vi "SeCrTS-DD Queue Data log module.vi"(8 "error in":errorcluster) -> (0 "error out":errorcluster)   [LabVIEW 2022 SP3]
uses:
  Control/SeCrTS-Datalog enumDD.ctl
  Globals/SeCrTS-DD globals.vi
panel:
  out "x":u32
  out "x-y":dbl
  out "Restart":bool
  out "Log health":bool
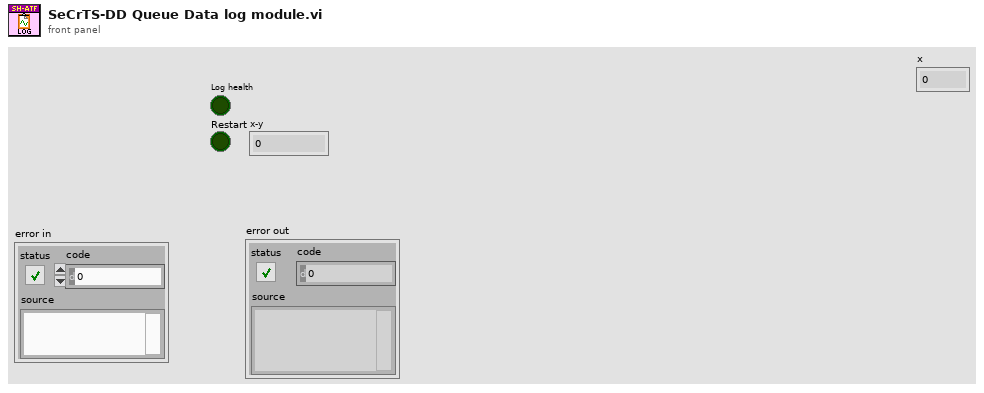
[diagram p1: front panel]
types:
  T1 = cluster{"Log In Progress?":bool, "Log Start Time":timestamp, "Analog Queues":refnum<queue>[], "Digital Queues":refnum<queue>[], "tdms file ref":refnum<k34>}
  T2 = typedef "SeCrTS-Datalog enumDD.ctl" = enum16{"Initialize", "Poll", "Create file", "log Analog", "log Digital", "Flush Queues", "Close file", "Error", "Exit"}
  T3 = enum16{"open", "open or create", "create or replace", "create", "open (read-only)"}
  T4 = cluster{"Datalog path":path, "Configuration path":path, "Signal list path":path, "Sub vi's":path, "Authentication":path}
  T5 = cluster{"Channel names":cluster{"AI_C_Data P":string[], "AI_V_Data P":string[], "AO_Data P":string[], "DO_Data P":string[], "ACC_Data P":string[], "TC Data P":string[], "Drive_A_C":string[], "Drive_A_D":string[], "AI_C_Data S":string[], "DO_Data S":string[]}, "DI Names":cluster{"Di P":string[], "Di S":string[]}}
  T6 = cluster{"AI_C_Data P":string[], "AI_V_Data P":string[], "AO_Data P":string[], "DO_Data P":string[], "ACC_Data P":string[], "TC Data P":string[], "Drive_A_C":string[], "Drive_A_D":string[], "AI_C_Data S":string[], "DO_Data S":string[]}
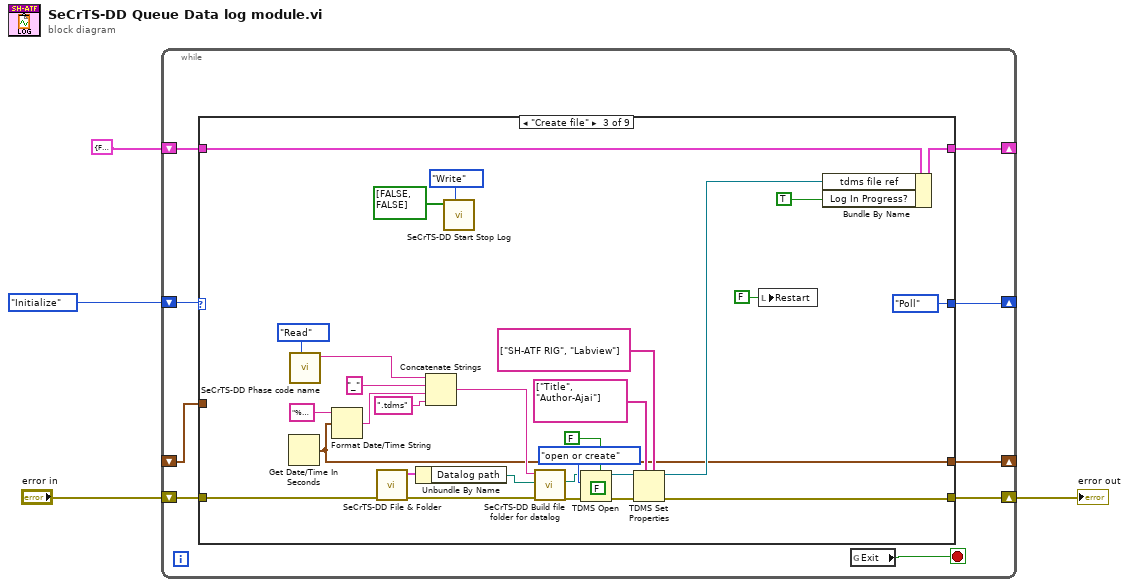
[diagram p0: block diagram]
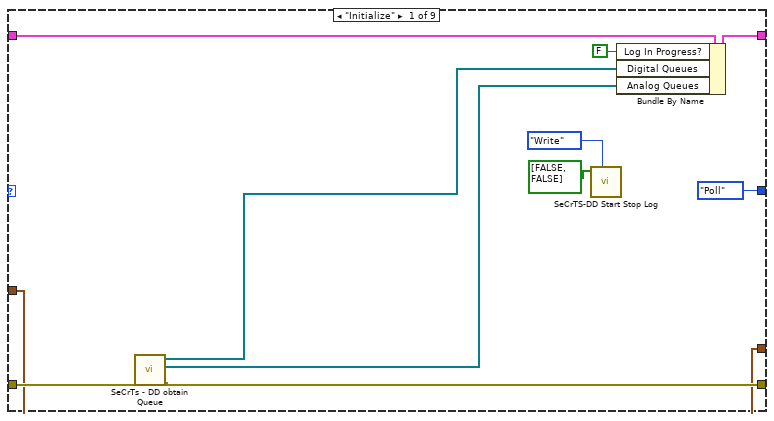
[diagram p2: hidden frame]
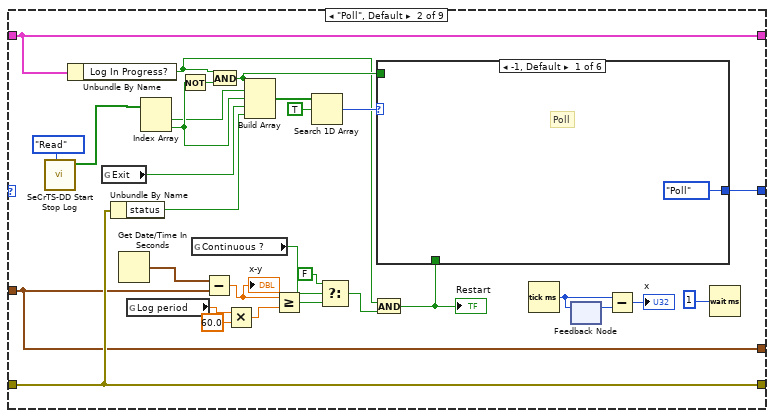
[diagram p3: hidden frame]
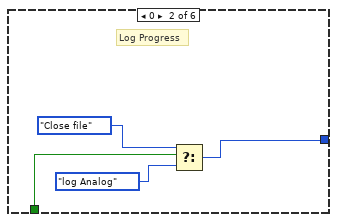
[diagram p4: hidden frame]
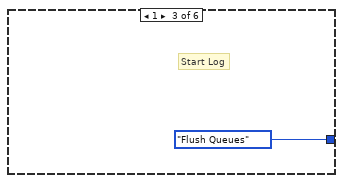
[diagram p5: hidden frame]
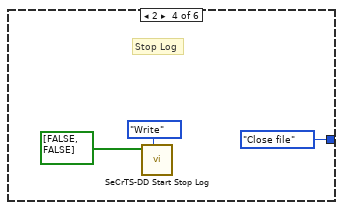
[diagram p6: hidden frame]
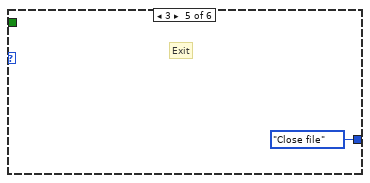
[diagram p7: hidden frame]
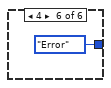
[diagram p8: hidden frame]
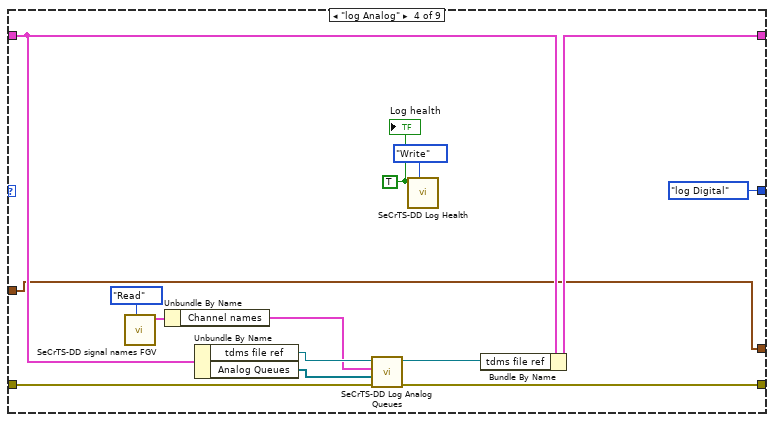
[diagram p9: hidden frame]
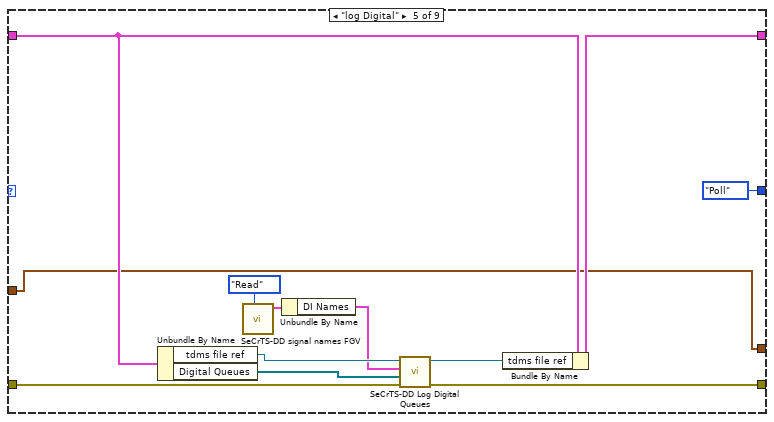
[diagram p10: hidden frame]
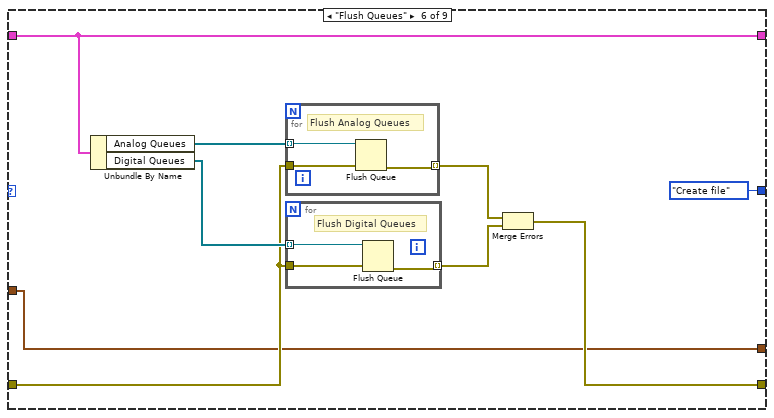
[diagram p11: hidden frame]
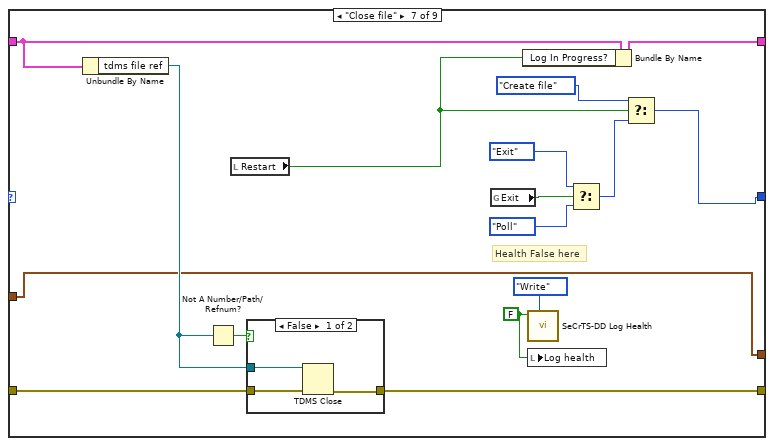
[diagram p12: hidden frame]
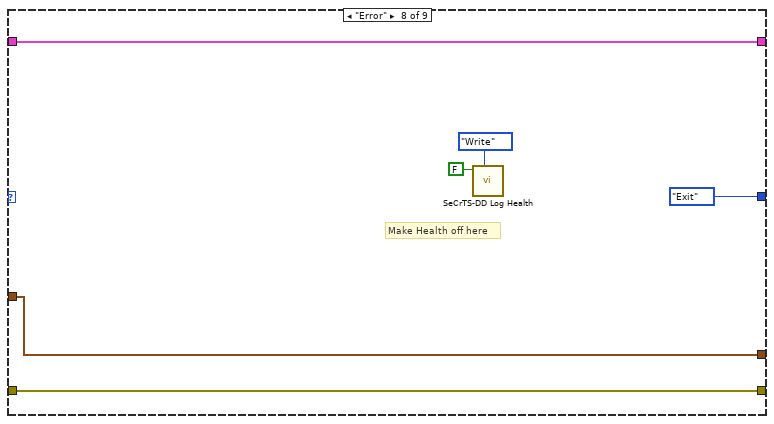
[diagram p14: hidden frame]
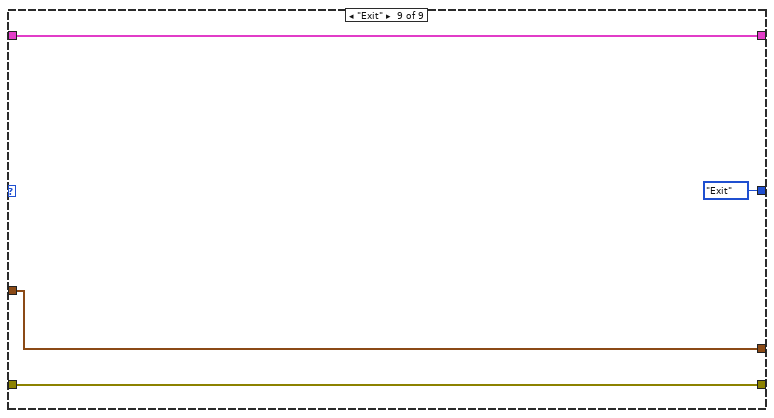
[diagram p15: hidden frame]
diagram:
  n1 = while {
    shift-right: [w8] -> _
    shift-left: SeCrTS-Datalog_enumDD."Initialize" -> [w13]
    shift-right: [w10] -> _
    shift-left: T1 {"Log In Progress?"=FALSE, "Log Start Time"=timestamp(0 s since 1904-01-01), "Analog Queues"=[], "Digital Queues"=[], "tdms file ref"=refnum} -> [w11]
    shift-right: [w9] -> w1
    shift-left: "error in" -> [w12]
    shift-right: [w5] -> _
    shift-left: _ -> [w6]
    stop <- w7 stop-if-true
    n2 = case shown="\"Create file\"" w13 {
      tunnel: w12 -> [w23 w48 w89 w105 w119 w125 w147 w159 w164]
      tunnel: w11 -> [w24 w54 w78 w107 w117 w128 w148 w161 w165]
      tunnel: [w22 w54 w77 w102 w114 w128 w149 w161 w165] -> w10
      tunnel: [w18 w48 w74 w104 w118 w122 w146 w159 w164] -> w9
      tunnel: [SeCrTS-Datalog_enumDD."Poll" w49 SeCrTS-Datalog_enumDD."Poll" SeCrTS-Datalog_enumDD."log Digital" SeCrTS-Datalog_enumDD."Poll" SeCrTS-Datalog_enumDD."Create file" w136 SeCrTS-Datalog_enumDD."Exit" SeCrTS-Datalog_enumDD."Exit"] -> w8
      tunnel: w6 -> [w16 w38 _ w95 w109 w121 w140 w156 w162]
      tunnel: [w16 w38 w68 w95 w109 w121 w140 w156 w162] -> w5
      frame "Initialize" {
        n3 = call "SeCrTs - DD obtain Queue.vi"("error in"=w23) -> ("error out"=w18:errorcluster, "AI_V_Data P\nAI_C_Data P\nAO_Data P\nDO_Data P\nACC_Data P\nTC Data P\nDrive_A_C \nDrive_A_D\nAI_C_Data S\nDO_Data S\nAI_V_Rms_P"=w19:refnum<queue>[], "DI P\nDI S"=w20:refnum<queue>[])  [unwired: 8 in]
        n4 = call "SeCrTS-DD Start Stop Log.vi"("Enum"=enum16{"Read", "Write"}."Write", "Start Stop log"=bool[] [FALSE, FALSE]) -> ()  [unwired: 8 in, 2 out]
        n5 = Bundle By Name(cluster=w24, "Log In Progress?"=FALSE, "Digital Queues"=w20, "Analog Queues"=w19) -> (w22:T1)
      }
      frame "Poll", Default {
        n6 = call "SeCrTS-DD Start Stop Log.vi"("Enum"=enum16{"Read", "Write"}."Read") -> ("Start Stop log R"=w34:bool[])  [unwired: 9 in, 1 out]
        n7 = Unbundle By Name(w54) -> ("Log In Progress?"=w28:bool)
        n8 = global read "SeCrTS-DD globals.vi" "Exit"() -> (w44:bool)
        n9 = Unbundle By Name(w48) -> ("status"=w53:bool)
        n10 = Get Date/Time In Seconds() -> (seconds since 1Jan1904=w40:timestamp)
        n11 = global read "SeCrTS-DD globals.vi" "Log period"() -> (w27:dbl)
        n12 = Index Array(array=w34) -> (element #1=w45:bool, element #2=w46:bool)  [unwired: 2 in]
        n13 = Not(x=w46) -> (.not. x?=w47:bool)
        n14 = global read "SeCrTS-DD globals.vi" "Continuous ?"() -> (w32:bool)
        n15 = Subtract(x=w40, y=w38) -> (x-y=w41:dbl)
        "x-y" <- w41
        n16 = And(x=w28, y=w47) -> (x .and. y?=w42:bool)
        n17 = Multiply(x=w27, y=60.0) -> (x*y=w25:dbl)
        n18 = Build Array(w42, w45, w46, w44, w53) -> (w52:bool[])
        n19 = Greater Or Equal?(x=w41, y=w25) -> (x >= y?=w31:bool)
        n20 = Search 1D Array(1D array=w52, element=TRUE) -> (index of element=w50:i32)  [unwired: 1 in]
        n21 = Select(t=FALSE, s=w32, f=w31) -> (s? t:f=w29:bool)
        n22 = And(x=w28, y=w29) -> (x .and. y?=w39:bool)
        "Restart" <- w39
        n23 = case shown="-1, Default" w50 {
          tunnel: [SeCrTS-Datalog_enumDD."Poll" w56 SeCrTS-Datalog_enumDD."Flush Queues" SeCrTS-Datalog_enumDD."Close file" SeCrTS-Datalog_enumDD."Close file" SeCrTS-Datalog_enumDD."Error"] -> w49
          tunnel: w42 -> [_ _ _ _ _ _]
          tunnel: w39 -> [_ w59 _ _ _ _]
          frame -1, Default {
            # "Poll"
          }
          frame 0 {
            # "Log Progress"
            n24 = Select(t=SeCrTS-Datalog_enumDD."Close file", s=w59, f=SeCrTS-Datalog_enumDD."log Analog") -> (s? t:f=w56:T2)
          }
          frame 1 {
            # "Start Log"
          }
          frame 2 {
            # "Stop Log"
            n25 = call "SeCrTS-DD Start Stop Log.vi"("Enum"=enum16{"Read", "Write"}."Write", "Start Stop log"=bool[] [FALSE, FALSE]) -> ()  [unwired: 8 in, 2 out]
          }
          frame 3 {
            # "Exit"
          }
          frame 4 {
          }
        }
        n26 = Tick Count (ms)() -> (millisecond timer value=w36:u32)
        n27 = feedback #1() -> (w37:u32)  [unwired: 1 in]
        n28 = feedback-in #1(w36) -> ()
        n29 = Subtract(x=w36, y=w37) -> (x-y=→"x":u32)
        n30 = Wait (ms)(milliseconds to wait=u32 1 ("millisecond timer value")) -> ()  [unwired: 1 out]
      }
      frame "Create file" {
        (unwired) FALSE ("disable buffering? (T)")
        n31 = Get Date/Time In Seconds() -> (seconds since 1Jan1904=w68:timestamp)
        n32 = call "SeCrTS-DD Phase code name.vi"("Enum"=enum16{"Read", "Write"}."Read") -> ("Phase codeR"=w69:string)  [unwired: 9 in, 1 out]
        n33 = Format Date/Time String(time format string (%c)="%Y_%b_%d_%Hh_%Mm_%Ssec", seconds (now)=w68) -> (date/time string=w94:string)  [unwired: 1 in]
        n34 = call "SeCrTS-DD File & Folder.vi"("error in (no error)"=w89) -> ("error out"=w88:errorcluster, "File Output"=w87:T4)  [unwired: 9 in]
        n35 = Unbundle By Name(w87) -> ("Datalog path"=w86:path)
        n36 = Concatenate Strings(w69, "_" ("string"), w94, ".tdms" ("string")) -> (w90:string)
        n37 = call "SeCrTS-DD Start Stop Log.vi"("Enum"=enum16{"Read", "Write"}."Write", "Start Stop log"=bool[] [FALSE, FALSE]) -> ()  [unwired: 8 in, 2 out]
        n38 = call "SeCrTS-DD Build file folder for datalog.vi"("error in (no error)"=w88, "Base Path"=w86, "File Name"=w90) -> ("error out"=w80:errorcluster, "Result File path"=w79:path)  [unwired: 6 in, 1 out]
        n39 = TDMS Open(5:FALSE ("create index file? (T)"), 8:w80, 10:T3."open or create" ("operation (0:open)"), 11:w79) -> (0:w84:errorcluster, 3:w83:refnum<k34>)  [unwired: 3 in]
        n40 = TDMS Set Properties(5:string[] ["SH-ATF RIG", "Labview"] ("property names"), 7:string[] ["Title", "Author-Ajai"] ("property names"), 8:w84, 11:w83) -> (0:w74:errorcluster, 3:w76:refnum<k34>)  [unwired: 4 out]
        n41 = local write "Restart"(FALSE ("Restart")) -> ()
        n42 = Bundle By Name(cluster=w78, "tdms file ref"=w76, "Log In Progress?"=TRUE) -> (w77:T1)
      }
      frame "log Analog" {
        w99 = TRUE ("Log health")
        n43 = call "SeCrTS-DD signal names FGV.vi"("Enum"=enum16{"Read", "Write"}."Read") -> ("Signal names"=w97:T5)  [unwired: 9 in, 1 out]
        n44 = Unbundle By Name(w97) -> ("Channel names"=w96:T6)
        n45 = Unbundle By Name(w107) -> ("tdms file ref"=w103:refnum<k34>, "Analog Queues"=w106:refnum<queue>[])
        n46 = call "SeCrTS-DD Log Analog Queues.vi"("error in"=w105, "AI_V_Data P\nAI_C_Data P\nAO_Data P\nDO_Data P\nACC_Data P\nTC Data P\nDrive_A_C \nDrive_A_D\nAI_C_Data S\nDO_Data S\nAI_V_Rms_P"=w106, "Channel names"=w96, "tdms file in"=w103) -> ("error out"=w104:errorcluster, "tdms ref out"=w101:refnum<k34>)  [unwired: 6 in]
        n47 = call "SeCrTS-DD Log Health.vi"("Enum"=enum16{"Read", "Write"}."Write", "Log health"=w99) -> ()  [unwired: 8 in, 2 out]
        n48 = Bundle By Name(cluster=w107, "tdms file ref"=w101) -> (w102:T1)
        "Log health" <- w99
      }
      frame "log Digital" {
        n49 = Unbundle By Name(w117) -> ("tdms file ref"=w116:refnum<k34>, "Digital Queues"=w115:refnum<queue>[])
        n50 = call "SeCrTS-DD signal names FGV.vi"("Enum"=enum16{"Read", "Write"}."Read") -> ("Signal names"=w111:T5)  [unwired: 9 in, 1 out]
        n51 = Unbundle By Name(w111) -> ("DI Names"=w110:cluster{"Di P":string[], "Di S":string[]})
        n52 = call "SeCrTS-DD Log Digital Queues.vi"("error in"=w119, "DI_queue"=w115, "DI Names 2"=w110, "tdms file in"=w116) -> ("error out"=w118:errorcluster, "tdms file out"=w113:refnum<k34>)  [unwired: 6 in]
        n53 = Bundle By Name(cluster=w117, "tdms file ref"=w113) -> (w114:T1)
      }
      frame "Flush Queues" {
        n54 = Unbundle By Name(w128) -> ("Analog Queues"=w127:refnum<queue>[], "Digital Queues"=w126:refnum<queue>[])
        n55 = for {
          tunnel: w127 -> [w135] mode=indexing
          tunnel: w125 -> [w134]
          tunnel: [w133] -> w124 mode=indexing
          # "Flush Analog Queues"
          n56 = Flush Queue(queue=w135, error in (no error)=w134) -> (error out=w133:errorcluster)  [unwired: 2 out]
        }
        n57 = for {
          tunnel: w126 -> [w132] mode=indexing
          tunnel: w125 -> [w131]
          tunnel: [w130] -> w123 mode=indexing
          # "Flush Digital Queues"
          n58 = Flush Queue(queue=w132, error in (no error)=w131) -> (error out=w130:errorcluster)  [unwired: 2 out]
        }
        n59 = Merge Errors(w124, w123) -> (w122:errorcluster)
      }
      frame "Close file" {
        w141 = FALSE ("Log health")
        # "Health False here"
        n60 = Unbundle By Name(w148) -> ("tdms file ref"=w144:refnum<k34>)
        n61 = Not A Number/Path/Refnum?(number/path/refnum=w144) -> (NaN/Path/Refnum?=w145:bool)
        n62 = local read "Restart"() -> (w139:bool)
        n63 = case shown="False" w145 {
          tunnel: w147 -> [w154 w155]
          tunnel: [w153 w155] -> w146
          tunnel: w144 -> [w152 _]
          frame False {
            n64 = TDMS Close(8:w154, 11:w152) -> (0:w153:errorcluster)  [unwired: 1 out]
          }
          frame True {
          }
        }
        n65 = global read "SeCrTS-DD globals.vi" "Exit"() -> (w142:bool)
        n66 = Bundle By Name(cluster=w148, "Log In Progress?"=w139) -> (w149:T1)
        n67 = call "SeCrTS-DD Log Health.vi"("Enum"=enum16{"Read", "Write"}."Write", "Log health"=w141) -> ()  [unwired: 8 in, 2 out]
        n68 = local write "Log health"(w141) -> ()
        n69 = Select(t=SeCrTS-Datalog_enumDD."Exit", s=w142, f=SeCrTS-Datalog_enumDD."Poll") -> (s? t:f=w137:T2)
        n70 = Select(t=SeCrTS-Datalog_enumDD."Create file", s=w139, f=w137) -> (s? t:f=w136:T2)
      }
      frame "Error" {
        # "Make Health off here"
        n71 = call "SeCrTS-DD Log Health.vi"("Enum"=enum16{"Read", "Write"}."Write", "Log health"=FALSE) -> ()  [unwired: 8 in, 2 out]
      }
      frame "Exit" {
      }
    }
    n72 = global read "SeCrTS-DD globals.vi" "Exit"() -> (w7:bool)
  }
  "error out" <- w1
